vi "Impedance_Sweep_Freq.vi"() -> ()   [LabVIEW 2020]
uses:
  <vilib>/Analysis/1siggen.llb/Ramp Pattern by Samples.vi
  <vilib>/Analysis/baseanly.llb/Mean (DBL).vi
  <vilib>/Analysis/NI_AALBase.lvlib
panel:
  in  "Current Ch":tag="Dev3/ai1"
  in  "Voltage Ch":tag="Dev3/ai0"
  in  "Output channels":tag="Dev3/ao0"
  in  "TriggerLine":tag="/Dev3/ao/StartTrigger"
  out "Real (Z) - AvgInput":dbl=0.483159362565652 format="%#_3p"
  out "Capacitance - AvgInput":dbl=-4.6875540145244966e-05 format="%#_3p"
  out "Inductance - AvgInput":dbl=5.4037341931629855e-06 format="%#_3p"
  out "Test Number":i32
  in  "Num Avg":i32=5
  out "Mean Phase":dbl format="%0.2f"
  out "Mean Mag":dbl format="%.4p"
  out "Phase Graph":cluster{dbl[], "Ramp Pattern":dbl[]}(graph)
  in  "amplitude":dbl=0.1 format="%0.2p"
  in  "SampRate":dbl=250000.0 format="%0.2f"
  in  "Test Time":dbl=1.0 format="%#_6p"
  out "Mag Graph":cluster{dbl[], "Ramp Pattern":dbl[]}(graph)
  in  "samples":i32=128
  in  "start":dbl format="%#.4p"
  in  "end freq":dbl=1.0 format="%#.4p"
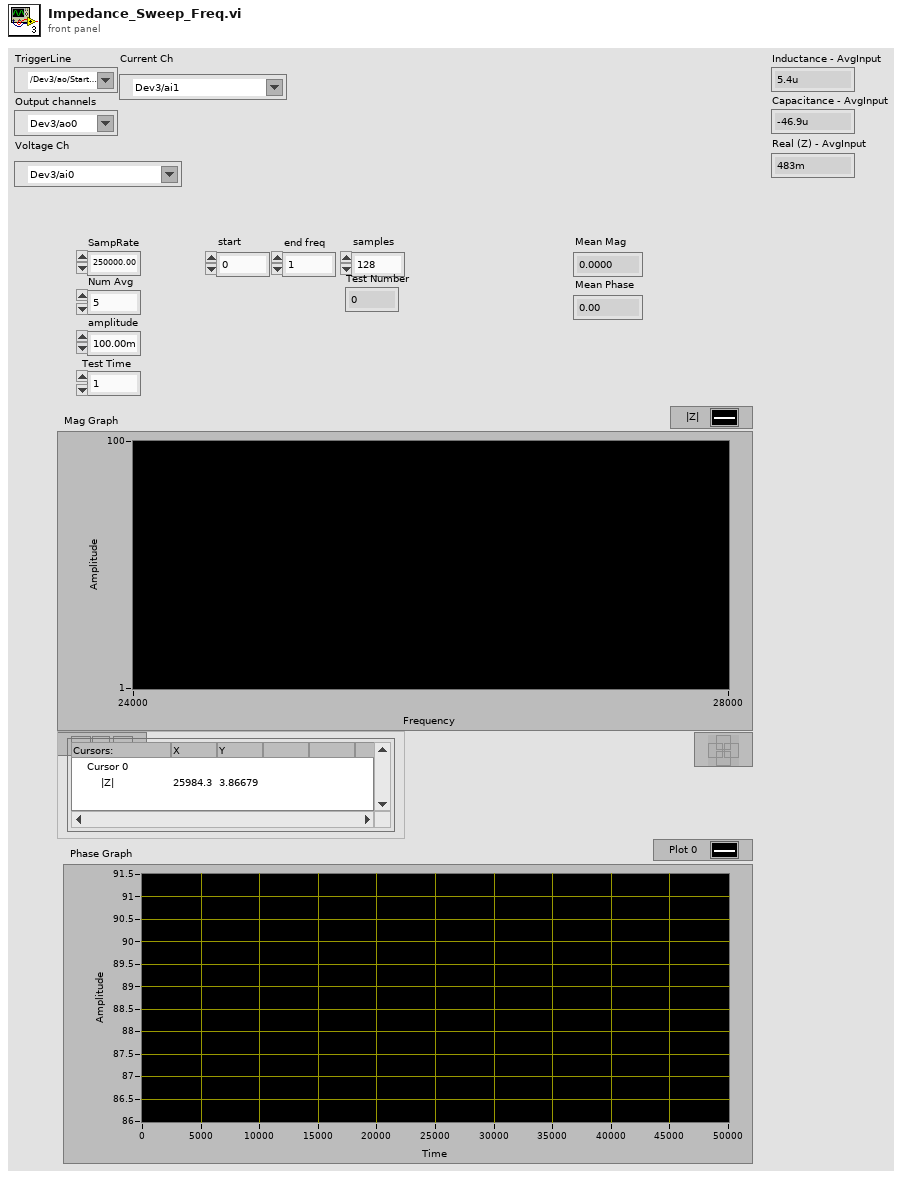
[diagram p1: front panel]
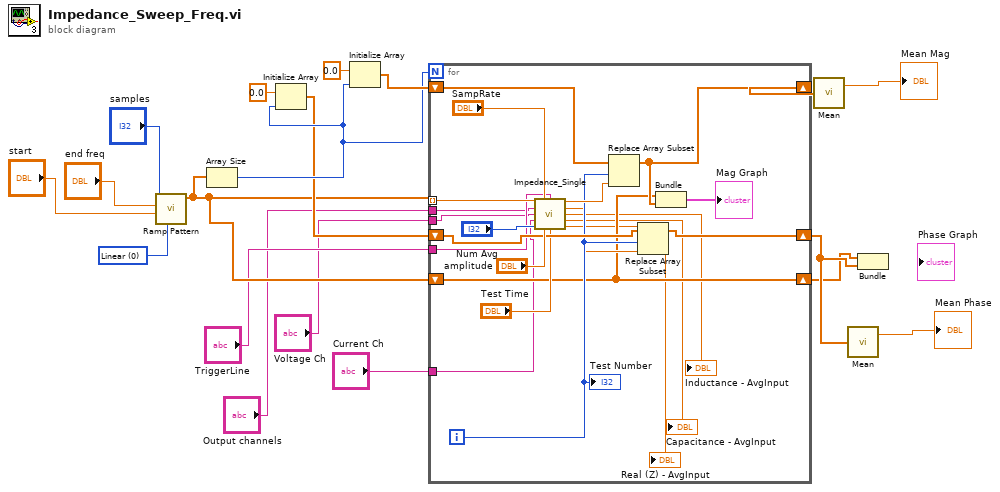
[diagram p0: block diagram]
diagram:
  w16 = u16 0 items=["Linear", "Logarithmic"] ("type")
  n1 = call-poly <vilib>:"Ramp Pattern.vi"("type"=w16, "start"="start", "end"="end freq", "samples"="samples") -> ("Ramp Pattern"=w7:dbl[])  [unwired: 6 in, 1 out]
  n2 = Array Size(array=w7) -> (size(s)=w12:i32)
  n3 = Initialize Array(0.0 ("element"), w12) -> (w11:dbl[])
  n4 = Initialize Array(0.0 ("element"), w12) -> (w14:dbl[])
  n5 = for {
    N: w12 -> [_]
    tunnel: w7 -> [w40] mode=indexing
    shift-right: [w28] -> w10
    shift-left: w14 -> [w39]
    shift-right: [w30] -> w6
    shift-left: w11 -> [w36]
    shift-right: [w27] -> w5
    shift-left: w7 -> [w27]
    tunnel: "TriggerLine" -> [w23]
    tunnel: "Output channels" -> [w22]
    tunnel: "Voltage Ch" -> [w21]
    tunnel: "Current Ch" -> [w20]
    i -> [w35]
    n6 = call "Impedance_Single.vi"("Measure Frequency"=w40, "Sampling Rate"="SampRate", "TriggerLine"=w23, "Output channels"=w22, "Voltage Ch"=w21, "Current Ch"=w20, "Number of runs"="Num Avg", "Amplitude (pk)"="amplitude", "Sampling Time"="Test Time") -> ("Impedance (Mag) - AvgInput"=w38:dbl, "Impedance (Phase) - AvgInput"=w34:dbl, "Inductance - AvgInput"=→"Inductance - AvgInput":dbl, "Capacitance - AvgInput"=→"Capacitance - AvgInput":dbl, "Real (Z) - AvgInput"=→"Real (Z) - AvgInput":dbl)  [unwired: 2 in]
    n7 = Replace Array Subset(array=w39, new element=w38, index=w35) -> (w28:dbl[])
    n8 = Replace Array Subset(array=w36, new element=w34, index=w35) -> (w30:dbl[])
    n9 = Bundle("Ramp Pattern"=w27, w28) -> (→"Mag Graph":cluster{"Ramp Pattern":dbl[], dbl[]})  [unwired: 1 in]
    "Test Number" <- w35
  }
  n10 = call-poly <vilib>:"Mean.vi"("X"=w10) -> ("mean"=→"Mean Mag":dbl)  [unwired: 1 out]
  n11 = call-poly <vilib>:"Mean.vi"("X"=w6) -> ("mean"=→"Mean Phase":dbl)  [unwired: 1 out]
  n12 = Bundle("Ramp Pattern"=w5, w6) -> ()  [unwired: 1 in, 1 out]
